vi "Swerve Rotate To Angle PID.vi"(6 "Target Cycle Time(S)":dbl=1.0 format="%.3f", 8 "PID Config":T3={"Gains"={"P"=1.0, "I"=0.01, "D"=0.0, "F"=0.0}, "Error Allowed"={"High"=0.1, "Low"=-0.1}, "I Zone"={"High"=10.0, "Low"=-10.0}, "Max Out"={"FWD"=100.0, "REV"=-100.0}, "Max I Accu"={"High"=0.0, "Low"=0.0}, "CL Ramp Rate (S)"=0.0} {"Max I Accu"."Low" format="%#.8f"; "Max I Accu"."High" format="%#.8f"; "Gains"."F" format="%#.8f"; "Gains"."D" format="%#.8f"; "Gains"."I" format="%#.8f"; "Gains"."P" format="%#.8f"; "Error Allowed"."Low" format="%#.8f"; "Error Allowed"."High" format="%#.8f"; "I Zone"."Low" format="%#.8f"; "I Zone"."High" format="%#.8f"; "Max Out"."REV" format="%.2f"; "Max Out"."FWD" format="%.2f"}, 9 "Current Yaw":T1 scale format="%.3f", 11 "Target Yaw":T1 scale format="%.3f") -> (0 "At Angle Out":bool, 1 "PROCESS Error Out":dbl, 3 "Direction.Rotate(Yaw) CCW 1 CW -1 Out":T2 scale=1.0..-1.0)   [LabVIEW 2020, in "SwerveDrive_ACT.lvlib"]
uses:
  SwerveDrive_ACT.lvlib
  Shared Code/TypeDefs/Cluster_PID Config.ctl
  Shared Code/TypeDefs/Cluster_PID Gains.ctl
  Shared Code/TypeDefs/Cluster_High-Low.ctl
  Shared Code/TypeDefs/Cluster_FWD  REV Values.ctl
  Type Defs/NUM_Rotate Input.ctl
  Shared Code/TypeDefs/Dial_Compase heading unit circle CCW positive.ctl
panel:
  out "I Accumulator":dbl
  out "Error Out":dbl
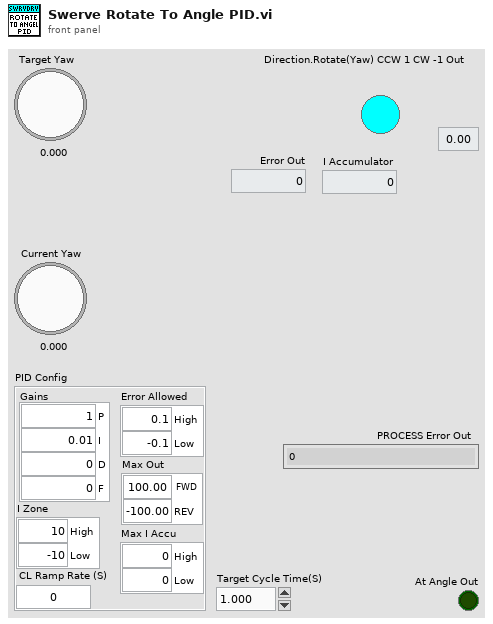
[diagram p1: front panel]
types:
  T1 = typedef "Dial_Compase heading unit circle CCW positive.ctl" = dbl
  T2 = typedef "NUM_Rotate Input.ctl" = dbl
  T3 = typedef "Cluster_PID Config.ctl" = cluster{"Gains":T4, "Error Allowed":T5, "I Zone":T5, "Max Out":T6, "Max I Accu":T5, "CL Ramp Rate (S)":dbl}
  T4 = typedef "Cluster_PID Gains.ctl" = cluster{"P":dbl, "I":dbl, "D":dbl, "F":dbl}
  T5 = typedef "Cluster_High-Low.ctl" = cluster{"High":dbl, "Low":dbl}
  T6 = typedef "Cluster_FWD  REV Values.ctl" = cluster{"FWD":dbl, "REV":dbl}
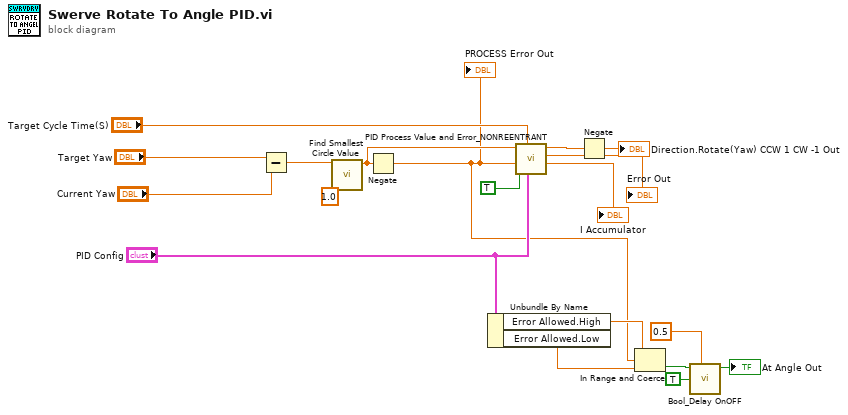
[diagram p0: block diagram]
diagram:
  n1 = Subtract(x="Target Yaw", y="Current Yaw") -> (x-y=w19:T1)
  n2 = call "Find Smallest Circle Value.vi"("Total Circle Value"=1.0, "Value"=w19) -> ("Smallest value on the circle"=w16:dbl)  [unwired: 9 in]
  n3 = Negate(x=w16) -> (-x=w7:dbl)
  "PROCESS Error Out" <- w7
  n4 = Unbundle By Name("PID Config") -> ("Error Allowed.High"=w13:dbl, "Error Allowed.Low"=w12:dbl)
  n5 = call "PID Process Value and Error_NONREENTRANT.vi"("PID Config"="PID Config", "Target Cycle Time(S)"="Target Cycle Time(S)", "Allowable Error Disables Accumulator"=TRUE, "ERROR"=w7, "Process Variable"=w16) -> ("I Accumulator"=→"I Accumulator":dbl, "Error Out"=→"Error Out":dbl, "Output Out"=w15:dbl)  [unwired: 2 in, 2 out]
  n6 = Negate(x=w15) -> (-x=→"Direction.Rotate(Yaw) CCW 1 CW -1 Out":dbl)
  n7 = In Range and Coerce(upper limit=w13, x=w7, lower limit=w12) -> (In Range?=w11:bool)  [unwired: 1 out]
  n8 = call "Bool_Delay OnOFF.vi"("Delay Time(S)"=0.5, "Delay On(t) Off(f)"=TRUE, "Input"=w11) -> ("Output"=→"At Angle Out":bool)  [unwired: 7 in, 1 out]
